vi "Read Element of Mission.vi"(8 "error in (no error)":errorcluster, 10 "index":i32, 11 "Load Mission Message in":refnum<class "Load Mission Message.lvclass">) -> (0 "error out":errorcluster, 2 "MissionOp":T1, 3 "Load Mission Message out":refnum<class "Load Mission Message.lvclass">)   [LabVIEW 2015, in "RDS Child Messages.lvlib" / "Load Mission Message.lvclass"]
uses:
  Load Mission Message.lvclass
  RDS Mission Controller Actor/MissionOp.ctl
  Load Mission Message.lvclass/Load Mission Message.ctl
  RDS Mission Controller Actor/RDS Mission Controller Actor.lvlib
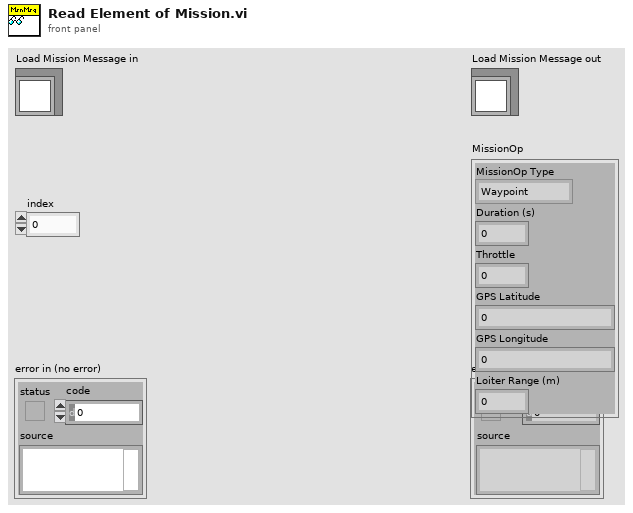
[diagram p1: front panel]
types:
  T1 = typedef "RDS Mission Controller Actor.lvlib/MissionOp.ctl" = cluster{"MissionOp Type":enum16{"Waypoint", "Loiter", "Wait", "Deploy AIP", "Stow AIP"}, "Duration (s)":dbl, "Throttle":dbl, "GPS Latitude":ext, "GPS Longitude":ext, "Loiter Range (m)":dbl}
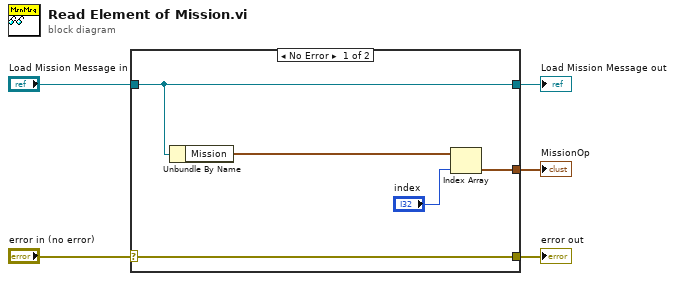
[diagram p0: block diagram]
diagram:
  n1 = case shown="No Error" "error in (no error)" {
    selector: "error in (no error)" -> [w10 w11]
    tunnel: [w10 w11] -> w4
    tunnel: [w9 w12] -> w2
    tunnel: "Load Mission Message in" -> [w9 w12]
    tunnel: [w6 _] -> w1
    frame No Error {
      n2 = Unbundle By Name(w9) -> ("Mission"=w8:T1[])
      n3 = Index Array(array=w8, index="index") -> (element=w6:T1)
    }
    frame Error {
    }
  }
  "error out" <- w4
  "Load Mission Message out" <- w2
  "MissionOp" <- w1
